vi "Salvar_txt.vi"(0 "path":path, 1 "Array":dbl[](array[numeric]), 2 "Array 2":dbl[](array[numeric]), 3 "Array 3":dbl[](array[numeric])) -> ()   [LabVIEW 2019]
uses:
  <vilib>/Utility/file.llb/Read Delimited Spreadsheet (string).vi
  <vilib>/Utility/file.llb/Write Delimited Spreadsheet (string).vi
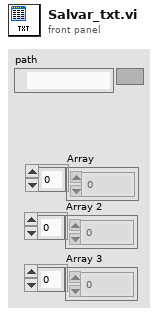
[diagram p1: front panel]
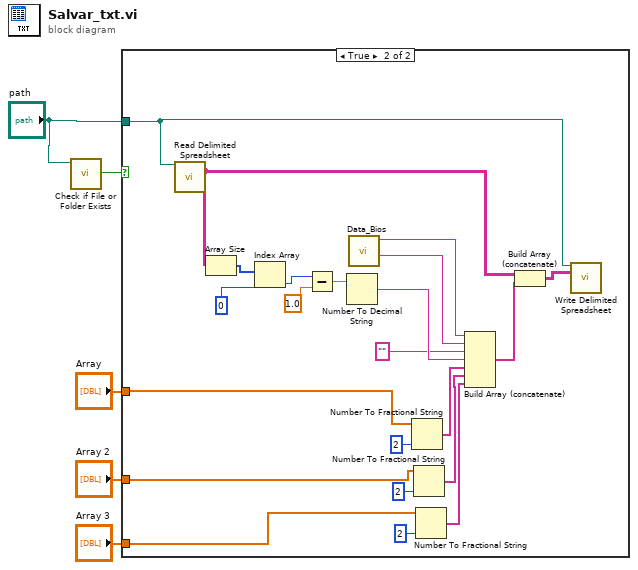
[diagram p0: block diagram]
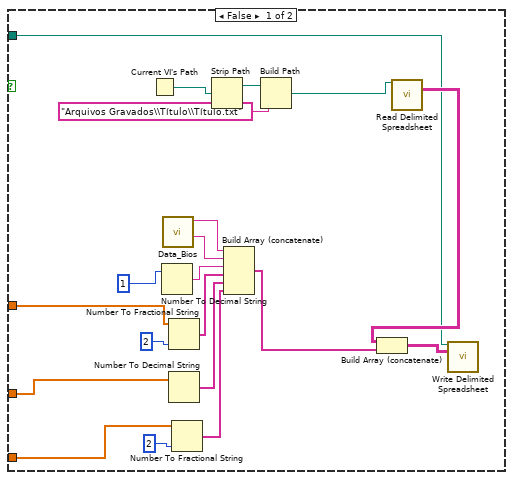
[diagram p2: hidden frame]
diagram:
  n1 = call <vilib>:"Check if File or Folder Exists.vi"("path"="path") -> ("file or folder exists?"=w1:bool)  [unwired: 8 in, 2 out]
  n2 = case shown="True" w1 {
    tunnel: "path" -> [w24 w45]
    tunnel: "Array" -> [w23 w36]
    tunnel: "Array 3" -> [w15 w33]
    tunnel: "Array 2" -> [w13 w31]
    frame False {
      n3 = Current VI's Path() -> (path=w10:path)
      n4 = Number To Decimal String(number=1) -> (decimal integer string=w20:string)  [unwired: 1 in]
      n5 = call "Data_Bios.vi"() -> ("Hora"=w6:string, "Data"=w7:string)  [unwired: 8 in, 1 out]
      n6 = Number To Fractional String(number=w23, precision (6)=i16 2) -> (F-format string=w22:string[])  [unwired: 2 in]
      n7 = Number To Decimal String(number=w13) -> (decimal integer string=w12:string[])  [unwired: 1 in]
      n8 = Number To Fractional String(number=w15, precision (6)=i16 2) -> (F-format string=w14:string[])  [unwired: 2 in]
      n9 = Strip Path(path=w10) -> (stripped path=w11:path)  [unwired: 1 out]
      n10 = Build Array (concatenate)(w7, w6, w20, w22, w12, w14) -> (w19:string[])
      n11 = Build Path(base path=w11, name or relative path="Arquivos Gravados\\Título\\Título.txt") -> (appended path=w8:path)
      n12 = call-poly <vilib>:"Read Delimited Spreadsheet.vi"("file path (dialog if empty)"=w8) -> ("all rows"=w25:string[][])  [unwired: 9 in, 5 out]
      n13 = Build Array (concatenate)(w25, w19) -> (w18:string[][])
      n14 = call-poly <vilib>:"Write Delimited Spreadsheet.vi"("file path (dialog if empty)"=w24, "2D data"=w18) -> ()  [unwired: 12 in, 2 out]
    }
    frame True {
      n15 = call-poly <vilib>:"Read Delimited Spreadsheet.vi"("file path (dialog if empty)"=w45) -> ("all rows"=w44:string[][])  [unwired: 9 in, 5 out]
      n16 = Array Size(array=w44) -> (size(s)=w47:i32[])
      n17 = Index Array(array=w47, index=0) -> (element=w38:i32)
      n18 = Subtract(x=w38, y=1.0) -> (x-y=w37:dbl)
      n19 = Number To Decimal String(number=w37) -> (decimal integer string=w43:string)  [unwired: 1 in]
      n20 = call "Data_Bios.vi"() -> ("Hora"=w28:string, "Data"=w29:string)  [unwired: 8 in, 1 out]
      n21 = Number To Fractional String(number=w36, precision (6)=i16 2) -> (F-format string=w42:string[])  [unwired: 2 in]
      n22 = Number To Fractional String(number=w31, precision (6)=i16 2) -> (F-format string=w30:string[])  [unwired: 2 in]
      n23 = Number To Fractional String(number=w33, precision (6)=i16 2) -> (F-format string=w32:string[])  [unwired: 2 in]
      n24 = Build Array (concatenate)(w29, w28, "" ("element"), w43, w42, w30, w32) -> (w41:string[])
      n25 = Build Array (concatenate)(w44, w41) -> (w40:string[][])
      n26 = call-poly <vilib>:"Write Delimited Spreadsheet.vi"("file path (dialog if empty)"=w45, "2D data"=w40) -> ()  [unwired: 12 in, 2 out]
    }
  }
